vi "filename_query_telem.vi"() -> (3 "appended array":string[][](array[string]))   [LabVIEW 2023]
panel:
  out "size(s)":i32
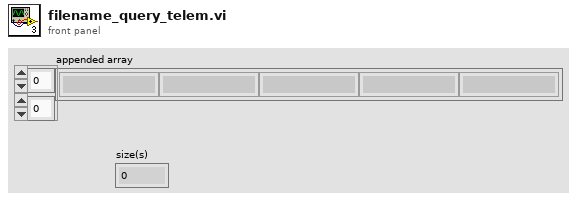
[diagram p1: front panel]
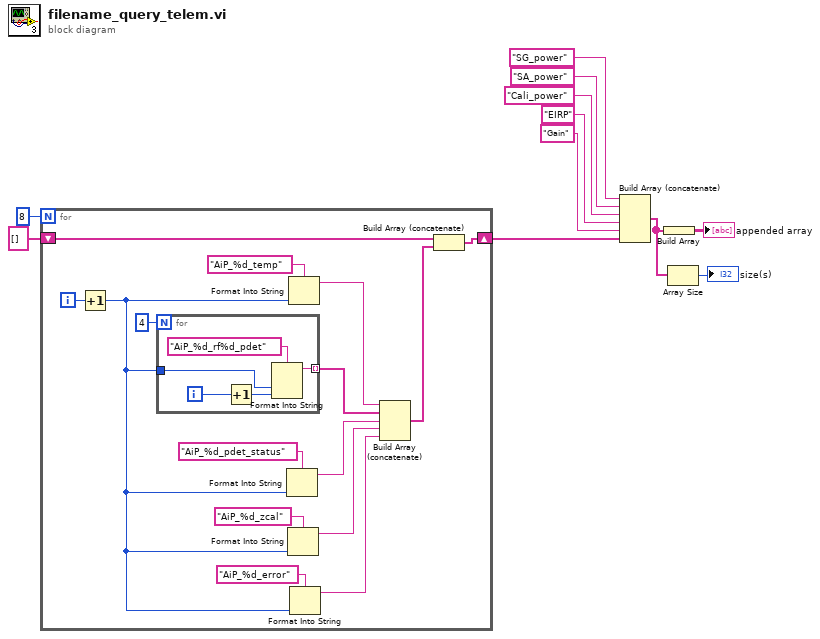
[diagram p0: block diagram]
diagram:
  n1 = for {
    N: 8 -> [_]
    shift-right: [w14] -> w8
    shift-left: string[] [] -> [w16]
    i -> [w13]
    n2 = Increment(x=w13) -> (x+1=w12:i32)
    n3 = for {
      N: 4 -> [_]
      tunnel: [w29] -> w20 mode=indexing
      tunnel: w12 -> [w27]
      i -> [w30]
      n4 = Increment(x=w30) -> (x+1=w28:i32)
      n5 = Format Into String(format string="AiP_%d_rf%d_pdet", w27, w28) -> (resulting string=w29:string)  [unwired: 2 in, 1 out]
    }
    n6 = Format Into String(format string="AiP_%d_pdet_status", w12) -> (resulting string=w19:string)  [unwired: 2 in, 1 out]
    n7 = Format Into String(format string="AiP_%d_zcal", w12) -> (resulting string=w18:string)  [unwired: 2 in, 1 out]
    n8 = Format Into String(format string="AiP_%d_temp", w12) -> (resulting string=w21:string)  [unwired: 2 in, 1 out]
    n9 = Format Into String(format string="AiP_%d_error", w12) -> (resulting string=w17:string)  [unwired: 2 in, 1 out]
    n10 = Build Array (concatenate)(w21, w20, w19, w18, w17) -> (w15:string[])
    n11 = Build Array (concatenate)(w16, w15) -> (w14:string[])
  }
  n12 = Build Array (concatenate)("SG_power" ("format string"), "SA_power" ("format string"), "Cali_power", "EIRP", "Gain", w8) -> (w6:string[])
  n13 = Build Array(w6) -> (→"appended array":string[][])
  n14 = Array Size(array=w6) -> (size(s)=→"size(s)":i32)
